vi "Handle Analog Command.vi"(8 "error in (no error)":errorcluster, 10 "Command":T1, 11 "DigitalControlModule in":refnum<class "DigitalControlModule.lvclass">) -> (0 "error out":errorcluster, 3 "DigitalControlModule out":refnum<class "DigitalControlModule.lvclass">)   [LabVIEW 2023, in "VolatusControl.lvlib" / "DigitalControlModule.lvclass"]
uses:
  DigitalControlModule.lvclass
  DigitalControlModule.lvclass/DigitalControlModule.ctl
  lv-vecto/Vecto/Group/Group.lvclass
  Volatus/Module/Module.lvclass
  lv-vecto/Vecto/Group DBL/Group DBL.lvclass
  C:/dev/volatus/mts-volatus-super/libs/lv-vecto/Vecto/Group/Group.lvclass
  C:/dev/volatus/mts-volatus-super/libs/lv-vecto/Vecto/Group DBL/Group DBL.lvclass
  C:/dev/volatus/mts-volatus-super/libs/lv-volatus/Volatus/Module/Module.lvclass
  C:/dev/volatus/mts-volatus-super/libs/lv-volatus/VolatusControl/DigitalControlModule/DigitalControlModule.lvclass
  messages/CmdAnalog/Data.ctl
  messages/CmdAnalog/CmdAnalog.lvlib
  messages/CmdAnalogMultiple/Data.ctl
  messages/CmdAnalogMultiple/CmdAnalogMultiple.lvlib
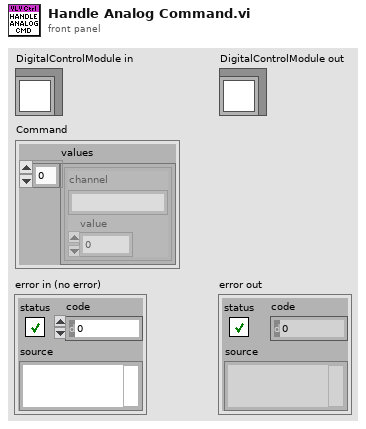
[diagram p1: front panel]
types:
  T1 = typedef "CmdAnalogMultiple.lvlib/Data.ctl" = cluster{"values":T2[]}
  T2 = typedef "CmdAnalog.lvlib/Data.ctl" = cluster{"channel":string, "value":dbl}
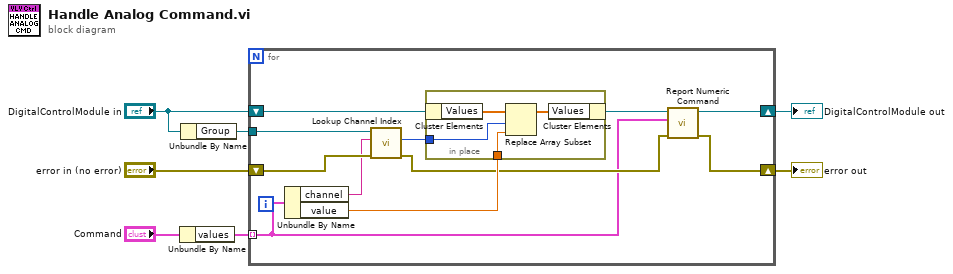
[diagram p0: block diagram]
diagram:
  n1 = Unbundle By Name("Command") -> ("values"=w1:T2[])
  n2 = Unbundle By Name("DigitalControlModule in") -> ("Group"=w7:refnum<class "Group DBL.lvclass">)
  n3 = for {
    tunnel: w7 -> [w17]
    shift-right: [w11] -> w5
    shift-left: "DigitalControlModule in" -> [w13]
    shift-right: [w9] -> w4
    shift-left: "error in (no error)" -> [w18]
    tunnel: w1 -> [w8] mode=indexing
    n4 = Unbundle By Name(w8) -> ("channel"=w16:string, "value"=w14:dbl)
    n5 = call "Lookup Channel Index.vi"("error in (no error)"=w18, "Channel Name"=w16, "Group in"=w17) -> ("error out"=w10:errorcluster, "Index"=w15:i32)  [unwired: 6 in, 1 out]
    n6 = in-place {
      in-place-border: w15 -> [w21]
      in-place-border: w14 -> [w20]
      n7 = in-place-cluster #1(w13) -> ("Values"=w22:dbl[])
      n8 = Replace Array Subset(array=w22, new element=w20, index=w21) -> (w19:dbl[])
      n9 = in-place-cluster #1("Values"=w19) -> (w12:refnum<class "DigitalControlModule.lvclass">)
    }
    n10 = call "Report Numeric Command.vi"("error in (no error)"=w10, "Command"=w8, "Module in"=w12) -> ("error out"=w9:errorcluster, "Module out"=w11:refnum<class "DigitalControlModule.lvclass">)  [unwired: 7 in]
  }
  "error out" <- w4
  "DigitalControlModule out" <- w5
